vi "Create.vi"(8 "error in (no error)":errorcluster, 11 "Project Path":path) -> (0 "error out":errorcluster, 3 "FlexWorktable out":refnum<class "FlexWorktable.lvclass">)   [LabVIEW 2024, in "FlexWorktable.lvclass"]
uses:
  FlexWorktable.lvclass
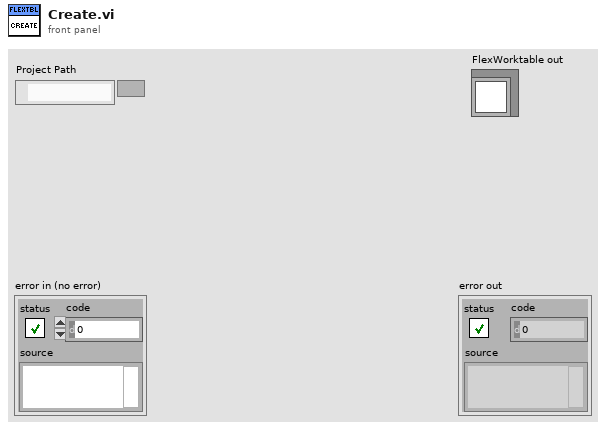
[diagram p1: front panel]
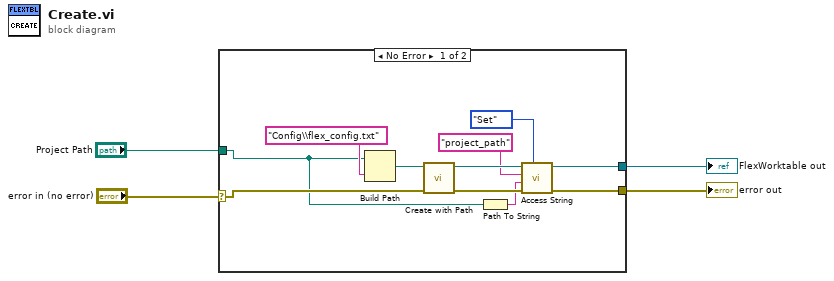
[diagram p0: block diagram]
diagram:
  n1 = case shown="No Error" "error in (no error)" {
    selector: "error in (no error)" -> [w13 w16]
    tunnel: [w10 w16] -> w3
    tunnel: [w5 _] -> w2
    tunnel: "Project Path" -> [w8 _]
    frame No Error {
      n2 = Build Path(base path=w8, name or relative path="Config\\flex_config.txt") -> (appended path=w14:path)
      n3 = call "Create with Path.vi"("error in (no error)"=w13, "flex_config path"=w14) -> ("error out"=w11:errorcluster, "FlexWorktable out"=w12:refnum<class "FlexWorktable.lvclass">)  [unwired: 8 in]
      n4 = Path To String(path=w8) -> (string=w6:string)
      n5 = call-dynamic "Access String.vi"("Get/Set"=enum16{"Get", "Set"}."Set", "error in (no error)"=w11, "Value in"=w6, "Key"="project_path", "FlexWorktable in"=w12) -> ("error out"=w10:errorcluster, "FlexWorktable out"=w5:refnum<class "FlexWorktable.lvclass">)  [unwired: 4 in, 1 out]
    }
    frame Error {
    }
  }
  "error out" <- w3
  "FlexWorktable out" <- w2
